vi "Find Class Path.vi"(8 "error in":errorcluster, 10 "Class Name":string, 11 "Config in":refnum<class "Config.lvclass">) -> (0 "error out":errorcluster, 2 "Class Path":path, 3 "Config out":refnum<class "Config.lvclass">)   [LabVIEW 2023, in "Config.lvlib" / "Config.lvclass"]
uses:
  Config.lvclass
  <vilib>/Utility/LVLibp/NI_PackedLibraryUtility.lvlib
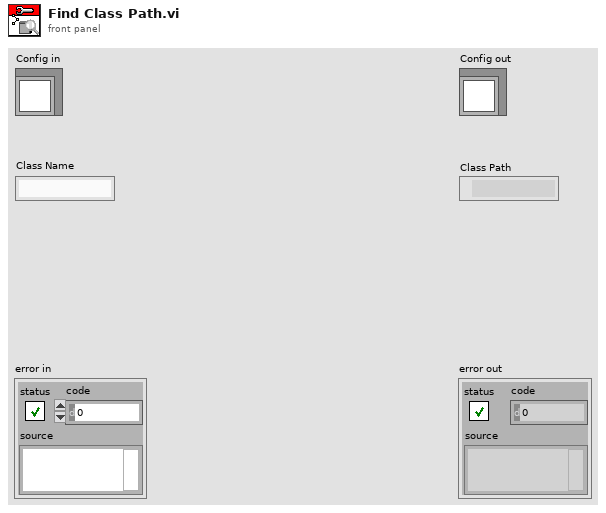
[diagram p1: front panel]
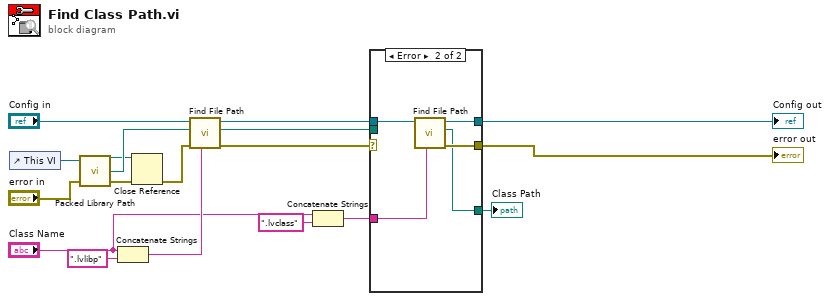
[diagram p0: block diagram]
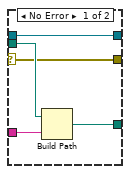
[diagram p2: hidden frame]
diagram:
  n1 = control-ref of="This VI"() -> (w6:refnum<vi>)
  n2 = call <vilib>:"Packed Library Path.vi"("error in (no error)"="error in", "vi reference"=w6) -> ("error out"=w3:errorcluster, "packed library path"=w5:path, "vi reference out"=w2:refnum<vi>)  [unwired: 1 in]
  n3 = Concatenate Strings("Class Name", ".lvlibp" ("string")) -> (w17:string)
  n4 = Close Reference(reference=w2, error in (no error)=w3) -> (error out=w1:errorcluster)
  n5 = call "Find File Path.vi"("File Name\nwith extension"=w17, "error in"=w1, "Path\n(Empty at top level)"=w5, "Config in"="Config in") -> ("error out"=w13:errorcluster, "File Path Control"=w11:path, "Config out"=w12:refnum<class "Config.lvclass">)  [unwired: 5 in]
  n6 = Concatenate Strings("Class Name", ".lvclass" ("string")) -> (w10:string)
  n7 = case shown="Error" w13 {
    selector: w13 -> [w19 _]
    tunnel: w12 -> [w20 w27]
    tunnel: w11 -> [w22 _]
    tunnel: w10 -> [w23 w25]
    tunnel: [w21 w24] -> w7
    tunnel: [w20 w26] -> w9
    tunnel: [w19 w28] -> w8
    frame No Error {
      n8 = Build Path(base path=w22, name or relative path=w23) -> (appended path=w21:path)
    }
    frame Error {
      n9 = call "Find File Path.vi"("File Name\nwith extension"=w25, "Config in"=w27) -> ("error out"=w28:errorcluster, "File Path Control"=w24:path, "Config out"=w26:refnum<class "Config.lvclass">)  [unwired: 7 in]
    }
  }
  "error out" <- w8
  "Config out" <- w9
  "Class Path" <- w7
